vi "Actor Core.vi"(8 "error in":errorcluster, 11 "Nested in":refnum<class "UI Actor.lvclass">) -> (0 "error out":errorcluster, 3 "Actor out":refnum<class "Actor.lvclass">)   [LabVIEW 2020, in "UI Actor.lvlib" / "UI Actor.lvclass"]
doc: "(<B>Filename</B>: Actor Framework.lvlib:Actor.lvclass:Actor Core.vi)\n\nReceives messages to the actor, reacts to them, and initiates any error handling that may shut the actor down.\n\nDescendant classes may override this VI to append parallel tasks for the actor to complete while it handles messages. Overrides use the Call Parent Method node."
uses:
  UI Actor.lvclass
  C:/Program Files (x86)/National Instruments/LabVIEW 2020/vi.lib/ActorFramework/Actor/Actor.lvclass
  <vilib>/ActorFramework/Actor/Actor.lvclass
  Coins/Coins.lvclass
  UI Actor.lvclass/UI Actor.ctl
  Coins/Coins.lvclass/Coins.ctl
  <vilib>/ActorFramework/Actor/Actor.lvclass/Actor.ctl
  <vilib>/ActorFramework/Message Enqueuer/Message Enqueuer.lvclass/Message Enqueuer.ctl
  Read Currency.vi
  Coins/Write Caller SubPanel.vi
  Coins/Write Currency.vi
  <vilib>/ActorFramework/Message Enqueuer/Init from Existing Queue.vi
  <vilib>/ActorFramework/Message Enqueuer/Enqueue.vi
  <vilib>/ActorFramework/Stop Msg/Stop Msg.lvclass
  C:/Program Files (x86)/National Instruments/LabVIEW 2020/vi.lib/ActorFramework/Message/Message.lvclass
  <vilib>/ActorFramework/Message Priority Queue/Priority Enqueue.vi
  <vilib>/ActorFramework/Message Enqueuer/Message Enqueuer.lvclass
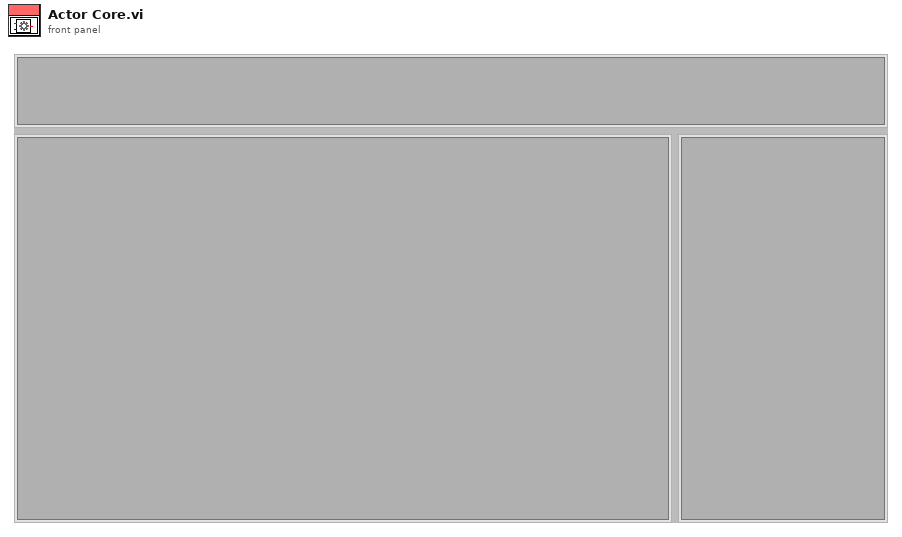
[diagram p1: front panel]
types:
  T1 = typedef "Currency Enum.ctl" = u16
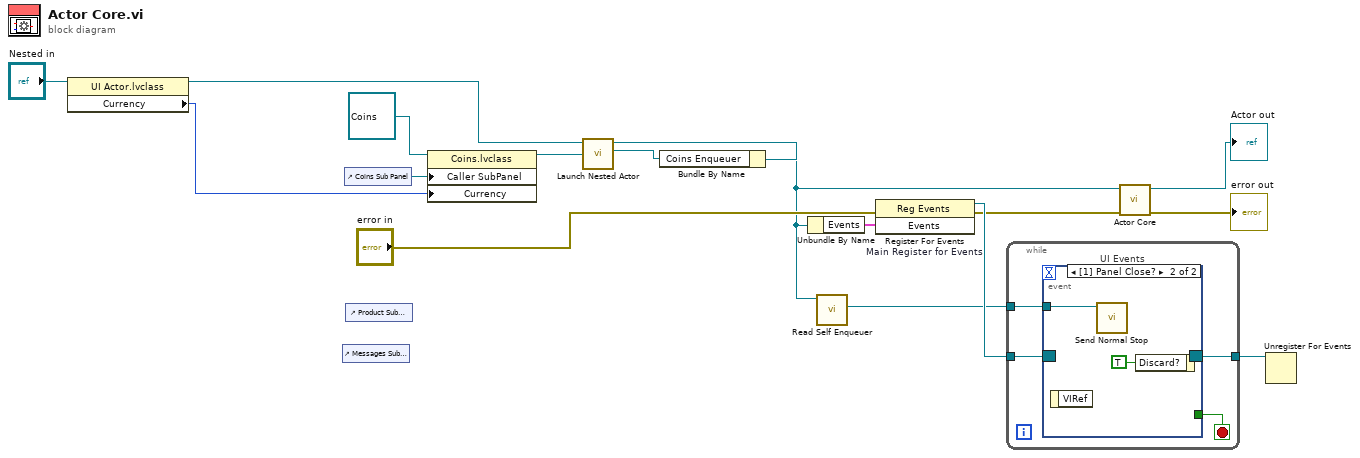
[diagram p0: block diagram]
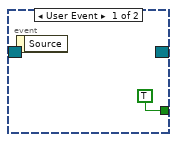
[diagram p2: hidden frame]
diagram:
  n1 = property class="UI Actor.lvclass"(reference="Nested in") -> (reference out=w2:refnum<class "UI Actor.lvclass">, "Currency"=w1:T1)  [unwired: 1 in, 1 out]
  n2 = control-ref of="Messages Sub Panel"() -> ()  [unwired: 1 out]
  n3 = control-ref of="Coins Sub Panel"() -> (w6:refnum<vi>)
  n4 = control-ref of="Product Sub Panel"() -> ()  [unwired: 1 out]
  n5 = property class="Coins.lvclass"(reference=refnum<class "Coins.lvclass"> refnum ("Coins.lvlib:Coins.lvclass"), "Caller SubPanel"=w6, "Currency"=w1) -> (reference out=w7:refnum<class "Coins.lvclass">)  [unwired: 1 in, 1 out]
  n6 = call <vilib>:"Launch Nested Actor.vi"("Nested Actor"=w7, "Caller Actor in"=w2) -> ("Nested Actor's Enqueuer"=w4:refnum<class "Message Enqueuer.lvclass">, "Caller Actor out"=w9:refnum<class "UI Actor.lvclass">)  [unwired: 7 in, 1 out]
  n7 = Bundle By Name(cluster=w9, "Coins Enqueuer"=w4) -> (w5:refnum<class "UI Actor.lvclass">)
  n8 = Unbundle By Name(w5) -> ("Events"=w14:cluster{"Stop":refnum<user-event>})
  n9 = call <vilib>:"Read Self Enqueuer.vi"("Actor"=w5) -> ("Self Enqueuer"=w12:refnum<class "Message Enqueuer.lvclass">)  [unwired: 10 in]
  n10 = register-events "Main Register for Events"(error in="error in", w14) -> (reference out=w15:refnum<event-registration>, error out=w10:errorcluster)  [unwired: 1 in]
  n11 = while {
    tunnel: w15 -> [w21]
    tunnel: [w19] -> w13
    tunnel: w12 -> [w18]
    stop <- w20 stop-if-true
    n12 = event "UI Events" shown="[1] Panel Close?" {
      selector: w21 -> [_ _]
      dyn-events: [_ _] -> w19
      timeout: _ -> [_ _]
      tunnel: [TRUE _] -> w20
      tunnel: w18 -> [_ w23]
      event User Event {
        n13 = event-data() -> ()  [unwired: 1 in, 1 out]
      }
      event Panel Close? {
        n14 = event-data() -> ()  [unwired: 1 in, 1 out]
        n15 = call <vilib>:"Send Normal Stop.vi"("Message Enqueuer"=w23) -> ()  [unwired: 10 in, 1 out]
        n16 = event-data("Discard?"=TRUE) -> ()  [unwired: 1 in, 1 out]
      }
    }
  }
  n17 = call-parent "Actor Core.vi"("error in"=w10, "Actor in"=w5) -> ("error out"=→"error out":errorcluster, "Actor out"=→"Actor out":refnum<class "Actor.lvclass">)  [unwired: 8 in]
  n18 = Unregister For Events(event registration refnum=w13) -> ()  [unwired: 1 in, 1 out]
